vi "api_mqttFree.vi"(8 "error in (no error)":errorcluster, 11 "mqtt in":refnum<class "mqtt.lvclass">) -> (0 "error out":errorcluster, 3 "mqtt out":refnum<class "mqtt.lvclass">)   [LabVIEW 2014, in "labview-mqtt.lvlib" / "mqtt.lvclass"]
uses:
  mqtt.lvclass
  mqtt.lvclass/mqtt.ctl
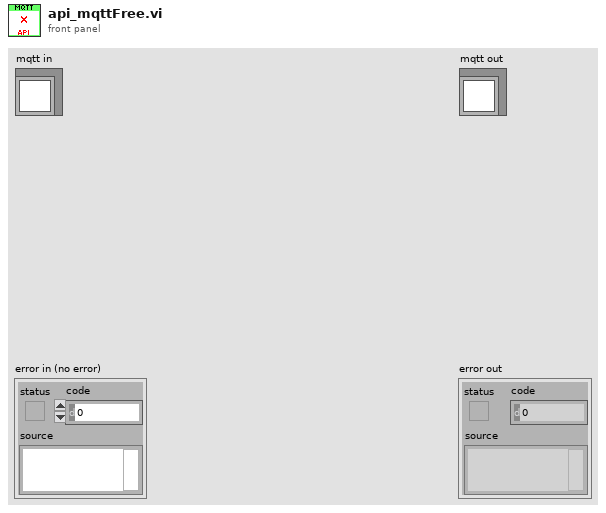
[diagram p1: front panel]
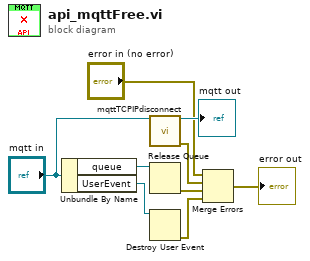
[diagram p0: block diagram]
diagram:
  n1 = Unbundle By Name("mqtt in") -> ("queue"=w9:refnum<queue>, "UserEvent"=w8:refnum<user-event>)
  n2 = call "mqttTCPIPdisconnect.vi"("mqtt in"="mqtt in") -> ("mqtt out"=→"mqtt out":refnum<class "mqtt.lvclass">, "error out"=w3:errorcluster)  [unwired: 13 in]
  n3 = Release Queue(queue=w9) -> (error out=w6:errorcluster)  [unwired: 2 in, 2 out]
  n4 = Destroy User Event(user event=w8) -> (error out=w7:errorcluster)  [unwired: 1 in]
  n5 = Merge Errors("error in (no error)", w3, w6, w7) -> (→"error out":errorcluster)
